vi "Generate Batches.vi"() -> ()   [LabVIEW 2020]
uses:
  <vilib>/Utility/file.llb/Read Delimited Spreadsheet (string).vi
  <vilib>/Utility/file.llb/Write Delimited Spreadsheet (string).vi
panel:
  out "subarray":string[][](array[string])
  in  "Parameters":T1={"Hours Predict"=1, "Hours to Skip"=1, "Previous Hours"=12, "Starting point"=0, "Predict Length"=12} {"Predict Length" min=1 step=1}
  in  "Batched Folder Extension":string="Time Series"
  out "error out":errorcluster
  in  "Number of Files":i32=10000
  out "Current Loop":i32=4988
  in  "Weather File Path":path=path "C:/Users/lukas/Documents/School/Ottawa/Work/Scintillometer/Scint Neural Network/TurbNet/TurbulentNetwork/All Weather Data MORE VARIABLES Scin No Interp Averaged.csv"
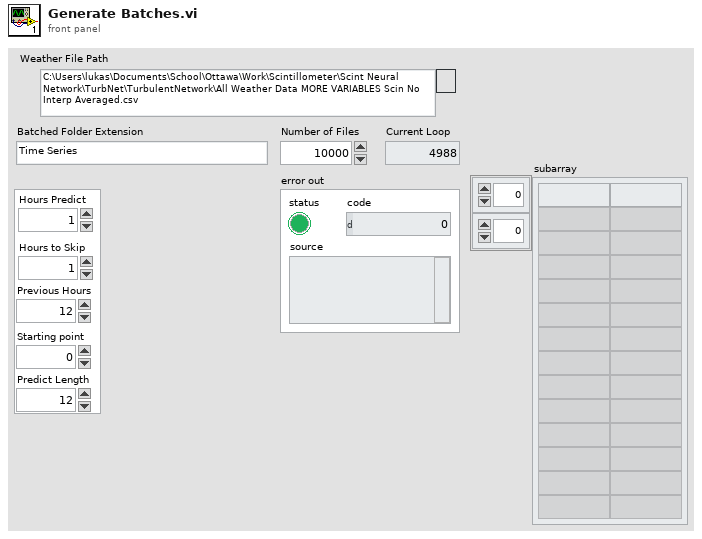
[diagram p1: front panel]
types:
  T1 = cluster{"Hours Predict":i32, "Hours to Skip":i32, "Previous Hours":i32, "Starting point":i32, "Predict Length":i32}
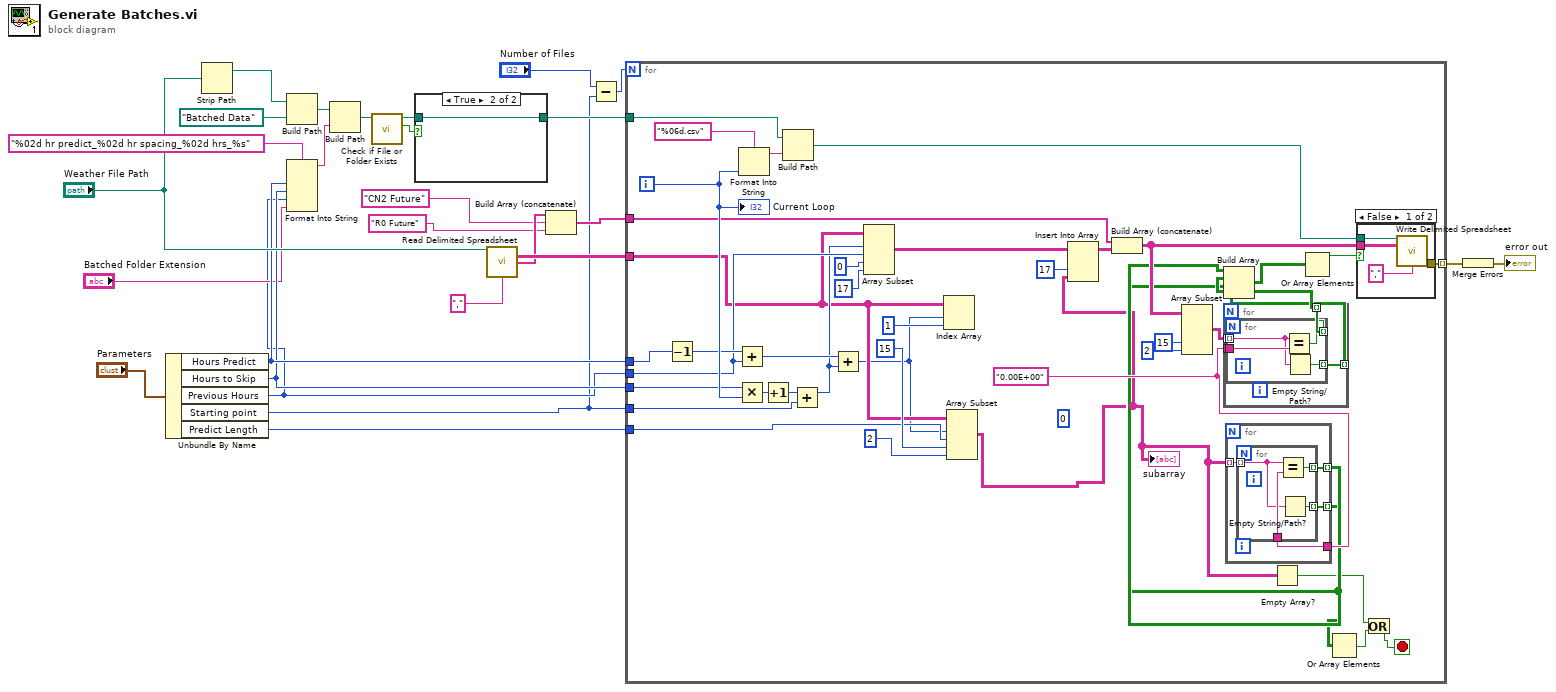
[diagram p0: block diagram]
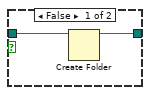
[diagram p2: hidden frame]
diagram:
  n1 = Unbundle By Name("Parameters") -> ("Hours Predict"=w9:i32, "Hours to Skip"=w8:i32, "Previous Hours"=w6:i32, "Starting point"=w3:i32, "Predict Length"=w2:i32)
  n2 = Strip Path(path="Weather File Path") -> (stripped path=w25:path)  [unwired: 1 out]
  n3 = Build Path(base path=w25, name or relative path=path "Batched Data") -> (appended path=w17:path)
  n4 = Format Into String(format string="%02d hr predict_%02d hr spacing_%02d hrs_%s", w9, w8, w6, "Batched Folder Extension") -> (resulting string=w11:string)  [unwired: 2 in, 1 out]
  n5 = Build Path(base path=w17, name or relative path=w11) -> (appended path=w16:path)
  n6 = call <vilib>:"Check if File or Folder Exists.vi"("path"=w16) -> ("file or folder exists?"=w15:bool, "dup path"=w14:path)  [unwired: 8 in, 1 out]
  n7 = case shown="True" w15 {
    tunnel: w14 -> [w29 w30]
    tunnel: [w28 w30] -> w13
    frame False {
      n8 = Create Folder(path (use dialog)=w29) -> (created path=w28:path)  [unwired: 2 in, 2 out]
    }
    frame True {
    }
  }
  n9 = call-poly <vilib>:"Read Delimited Spreadsheet.vi"("file path (dialog if empty)"="Weather File Path", "delimiter (\\t)"="," ("delimiter (\\t)")) -> ("all rows"=w23:string[][], "first row"=w20:string[])  [unwired: 8 in, 4 out]
  n10 = Build Array (concatenate)(w20, "CN2 Future" ("delimiter (\\t)"), "R0 Future" ("delimiter (\\t)")) -> (w18:string[])
  n11 = Subtract(x="Number of Files", y=w3) -> (x-y=w4:i32)
  n12 = for {
    N: w4 -> [_]
    tunnel: w23 -> [w41]
    tunnel: w13 -> [w67]
    tunnel: [w60] -> w22 mode=indexing
    tunnel: w18 -> [w59]
    tunnel: w9 -> [w55]
    tunnel: w8 -> [w54]
    tunnel: w6 -> [w53]
    tunnel: w3 -> [w44]
    tunnel: w2 -> [w40]
    i -> [w69]
    stop <- w31 stop-if-true
    (unwired) 0 ("index (row)")
    w38 = "0.00E+00" ("y")
    n13 = Decrement(x=w55) -> (x-1=w56:i32)
    n14 = Add(x=w56, y=w53) -> (x+y=w61:i32)
    n15 = Multiply(x=w54, y=w69) -> (x*y=w70:i32)
    n16 = Format Into String(format string="%06d.csv", w69) -> (resulting string=w66:string)  [unwired: 2 in, 1 out]
    n17 = Increment(x=w70) -> (x+1=w64:i32)
    n18 = Build Path(base path=w67, name or relative path=w66) -> (appended path=w65:path)
    n19 = Add(x=w64, y=w44) -> (x+y=w45:i32)
    n20 = Add(x=w61, y=w45) -> (x+y=w39:i32)
    n21 = Array Subset(array=w41, index (row)=w45, length (row)=w53, index (col)=0 ("index 2"), length (col)=17 ("length 2")) -> (w63:string[][])
    n22 = Index Array(array=w41, index (row)=w39, index (col)=1 ("disabled index (col)")) -> ()  [unwired: 1 out]
    n23 = Array Subset(array=w41, index (row)=w39, length (row)=w40, index (col)=15 ("disabled index (col)"), length (col)=2 ("length")) -> (w34:string[][])
    "subarray" <- w34
    n24 = Insert Into Array(array=w63, index (col)=17 ("disabled index (col)"), new element=w34) -> (w58:string[][])  [unwired: 1 in]
    n25 = Build Array (concatenate)(w59, w58) -> (w52:string[][])
    n26 = Array Subset(array=w52, index (col)=15 ("index"), length (col)=2 ("length")) -> (w49:string[][])  [unwired: 2 in]
    n27 = for {
      tunnel: w49 -> [w88] mode=indexing
      tunnel: [w87] -> w47 mode=indexing
      tunnel: w38 -> [w86]
      tunnel: [w85] -> w35 mode=indexing
      n28 = for {
        tunnel: w88 -> [w90] mode=indexing
        tunnel: [w92] -> w87 mode=indexing
        tunnel: w86 -> [w91]
        tunnel: [w89] -> w85 mode=indexing
        n29 = Equal?(x=w90, y=w91) -> (x = y?=w92:bool)
        n30 = Empty String/Path?(string/path=w90) -> (empty?=w89:bool)
      }
    }
    n31 = for {
      tunnel: w34 -> [w76] mode=indexing
      tunnel: w38 -> [w75]
      tunnel: [w74] -> w37 mode=indexing
      tunnel: [w73] -> w36 mode=indexing
      n32 = for {
        tunnel: w76 -> [w78] mode=indexing
        tunnel: w75 -> [w79]
        tunnel: [w80] -> w74 mode=indexing
        tunnel: [w77] -> w73 mode=indexing
        n33 = Equal?(x=w78, y=w79) -> (x = y?=w80:bool)
        n34 = Empty String/Path?(string/path=w78) -> (empty?=w77:bool)
      }
    }
    n35 = Build Array(w37, w47, w36, w35) -> (w46:bool[][][])
    n36 = Empty Array?(array=w34) -> (empty?=w32:bool)
    n37 = Or Array Elements(Boolean array=w46) -> (logical OR=w48:bool)
    n38 = Or Array Elements(Boolean array=w36) -> (logical OR=w33:bool)
    n39 = case shown="False" w48 {
      tunnel: w65 -> [w84 _]
      tunnel: [w82 _] -> w60
      tunnel: w52 -> [w81 _]
      frame False {
        n40 = call-poly <vilib>:"Write Delimited Spreadsheet.vi"("file path (dialog if empty)"=w84, "2D data"=w81, "delimiter (\\t)"="," ("delimiter (\\t)")) -> ("error out"=w82:errorcluster)  [unwired: 11 in, 1 out]
      }
      frame True {
      }
    }
    n41 = Or(x=w32, y=w33) -> (x .or. y?=w31:bool)
    "Current Loop" <- w69
  }
  n42 = Merge Errors(w22) -> (→"error out":errorcluster)
